vi "getSwitchOffTemperature.vi"(8 "error in (no error)":errorcluster, 11 "AndorIKonTempController in":refnum<class "AndorIKonTempController.lvclass">) -> (0 "error out":errorcluster, 2 "Switch Off Temperature":dbl=10.0, 3 "AndorIKonTempController out":refnum<class "AndorIKonTempController.lvclass">)   [LabVIEW 2011, in "Hardware.lvlib" / "Channels.lvlib" / "AndorIKonTempController.lvclass"]
uses:
  AndorIKonTempController.lvclass
  AndorIKonTempController.lvclass/AndorIKonTempController.ctl
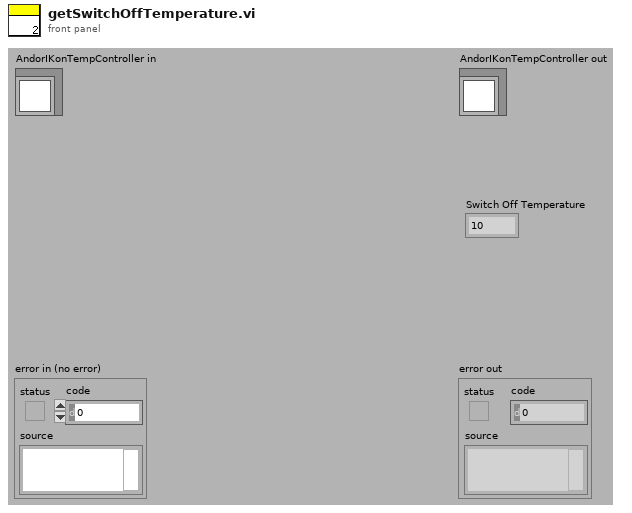
[diagram p1: front panel]
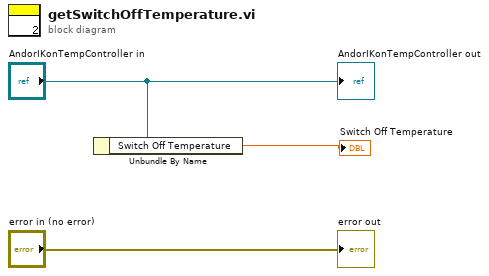
[diagram p0: block diagram]
diagram:
  n1 = Unbundle By Name("AndorIKonTempController in") -> ("Switch Off Temperature"=→"Switch Off Temperature":dbl)
  "error out" <- "error in (no error)"
  "AndorIKonTempController out" <- "AndorIKonTempController in"
